vi "Hex to  U16 NEW.vi"(10 "Numeric":i32, 11 "字符串":string="\u0000\u0000œ@") -> (3 "Vaule out":u16[](array[numeric]))   [LabVIEW 2017]
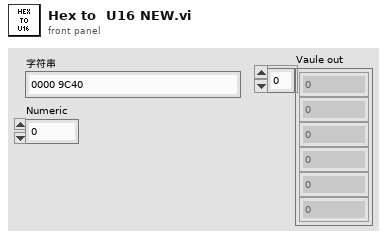
[diagram p1: front panel]
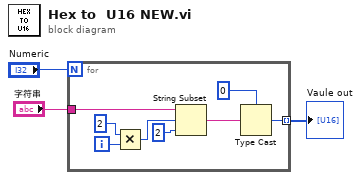
[diagram p0: block diagram]
diagram:
  n1 = for {
    N: "Numeric" -> [_]
    tunnel: "字符串" -> [w11]
    tunnel: [w4] -> w3 mode=indexing
    i -> [w7]
    n2 = Multiply(x=2, y=w7) -> (x*y=w8:i32)
    n3 = String Subset(string=w11, offset (0)=w8, length (rest)=2 ("length (rest)")) -> (substring=w6:string)
    n4 = Type Cast(type=u16 0 ("default (0 U32)"), x=w6) -> (*(type *) &x=w4:u16)
  }
  "Vaule out" <- w3
